vi "No Release Notifier Error.vi"(7 "error in":errorcluster) -> (8 "error out":errorcluster)   [LabVIEW 2020]
doc: "No Time Out Error.vi checks if a connection timed out error occurred and resets it to no error."
panel:
  # "Timeout is not an error."
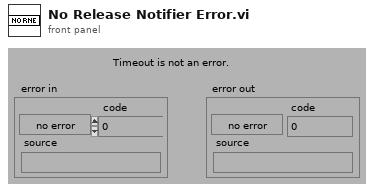
[diagram p1: front panel]
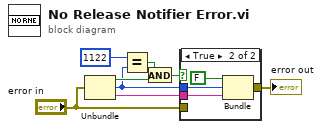
[diagram p0: block diagram]
diagram:
  n1 = Unbundle("error in") -> ("status"=w7:bool, "code"=w4:i32, "source"=w2:string)
  n2 = Equal?(x=1122, y=w4) -> (x = y?=w8:bool)
  n3 = And(x=w8, y=w7) -> (x .and. y?=w6:bool)
  n4 = case shown="True" w6 {
    tunnel: "error in" -> [w9 _]
    tunnel: w4 -> [_ w11]
    tunnel: [w9 w13] -> w3
    tunnel: w2 -> [_ w12]
    frame False {
    }
    frame True {
      n5 = Bundle(FALSE, "code"=w11, "source"=w12) -> (w13:cluster{bool, "code":i32, "source":string})  [unwired: 1 in]
    }
  }
  "error out" <- w3
